vi "del_avg_Qs.vi"(7 "avg_Q_data":T1) -> (8 "error out":errorcluster)   [LabVIEW 2023]
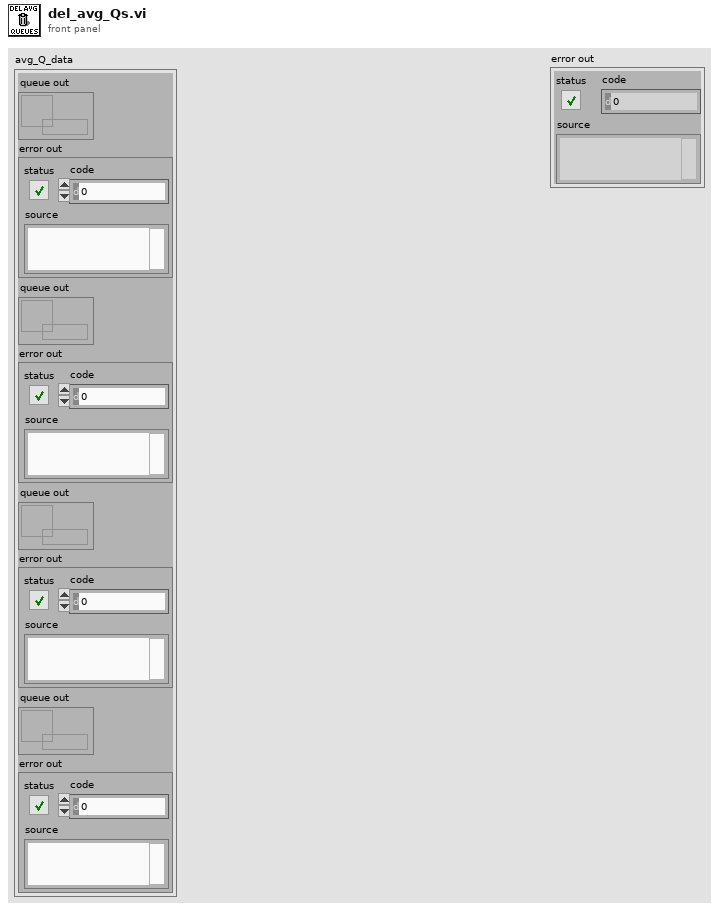
[diagram p1: front panel]
types:
  T1 = cluster{"queue out":refnum<queue>, "error out":errorcluster, "queue out":refnum<queue>, "error out":errorcluster, "queue out":refnum<queue>, "error out":errorcluster, "queue out":refnum<queue>, "error out":errorcluster}
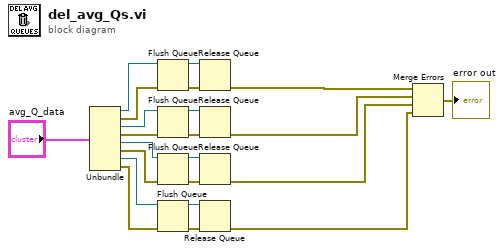
[diagram p0: block diagram]
diagram:
  n1 = Unbundle("avg_Q_data") -> ("queue out"=w22:refnum<queue>, "error out"=w21:errorcluster, "queue out"=w12:refnum<queue>, "error out"=w11:errorcluster, "queue out"=w10:refnum<queue>, "error out"=w9:errorcluster, "queue out"=w8:refnum<queue>, "error out"=w7:errorcluster)
  n2 = Flush Queue(queue=w22, error in (no error)=w21) -> (queue out=w20:refnum<queue>, error out=w19:errorcluster)  [unwired: 1 out]
  n3 = Flush Queue(queue=w12, error in (no error)=w11) -> (queue out=w18:refnum<queue>, error out=w17:errorcluster)  [unwired: 1 out]
  n4 = Flush Queue(queue=w10, error in (no error)=w9) -> (queue out=w16:refnum<queue>, error out=w15:errorcluster)  [unwired: 1 out]
  n5 = Flush Queue(queue=w8, error in (no error)=w7) -> (queue out=w14:refnum<queue>, error out=w13:errorcluster)  [unwired: 1 out]
  n6 = Release Queue(queue=w20, error in (no error)=w19) -> (error out=w6:errorcluster)  [unwired: 1 in, 2 out]
  n7 = Release Queue(queue=w18, error in (no error)=w17) -> (error out=w5:errorcluster)  [unwired: 1 in, 2 out]
  n8 = Release Queue(queue=w16, error in (no error)=w15) -> (error out=w4:errorcluster)  [unwired: 1 in, 2 out]
  n9 = Release Queue(queue=w14, error in (no error)=w13) -> (error out=w3:errorcluster)  [unwired: 1 in, 2 out]
  n10 = Merge Errors(w6, w5, w4, w3) -> (→"error out":errorcluster)
